vi "MechanicalActions.vi"() -> ()   [LabVIEW 2020]
panel:
  in  "stop":bool
  out "Cnt":u16
  in  "OK Button":bool
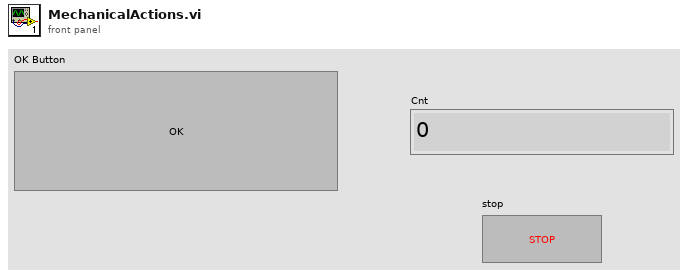
[diagram p1: front panel]
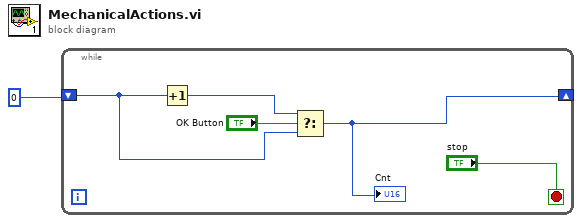
[diagram p0: block diagram]
diagram:
  n1 = while {
    shift-right: [w3] -> _
    shift-left: u16 0 ("Cnt") -> [w4]
    stop <- "stop" stop-if-true
    n2 = Increment(x=w4) -> (x+1=w5:u16)
    n3 = Select(t=w5, s="OK Button", f=w4) -> (s? t:f=w3:u16)
    "Cnt" <- w3
  }
